vi "Initialise.vi"(8 "error in (no error)":errorcluster, 11 "SMP in":refnum<class "SMP.lvclass">) -> (0 "error out":errorcluster, 3 "SMP out":refnum<class "SMP.lvclass">)   [LabVIEW 2013, in "SMP.lvclass"]
doc: "Initialise a new SMP object. This can be used to easily implement the Pipe and Filter design pattern within a state machine. The SMP object uses a queue internally.\n\nClick on <b>Detailed help</b> for a description of the Pipe and Filter design pattern.\n\n<b>SMP in: </b>If an existing SMP object is wired to the input, it will be closed upon the successfull initialisation of the new object. If the initialisation of the new object fails, the input object will be returned unchanged."
uses:
  SMP.lvclass
  private/classData.ctl
  Data types/operation.ctl
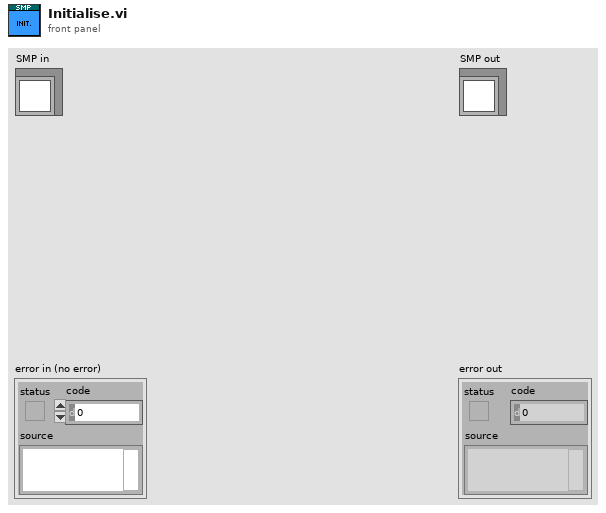
[diagram p1: front panel]
types:
  T1 = typedef "SMP.lvclass/operation.ctl" = cluster{"Name":string, "Data":variant}
  T2 = typedef "SMP.lvclass/classData.ctl" = cluster{"Q ref":refnum<queue>, "Previous data":variant, "Current pipe":T1[]}
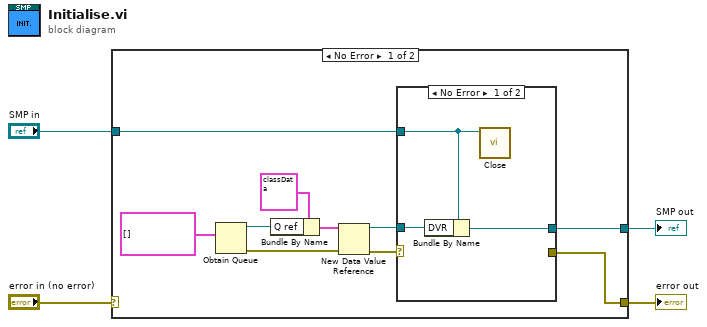
[diagram p0: block diagram]
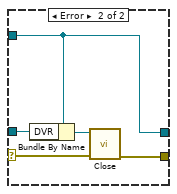
[diagram p2: hidden frame]
diagram:
  n1 = case shown="No Error" "error in (no error)" {
    selector: "error in (no error)" -> [_ w24]
    tunnel: [w5 w24] -> w3
    tunnel: [w6 w23] -> w1
    tunnel: "SMP in" -> [w8 w23]
    frame No Error {
      n2 = Obtain Queue(element data type=T1[] []) -> (queue out=w12:refnum<queue>, error out=w10:errorcluster)  [unwired: 4 in, 1 out]
      n3 = Bundle By Name(cluster=T2 {"Q ref"=refnum, "Previous data"=variant, "Current pipe"=[]} ("Class data"), "Q ref"=w12) -> (w11:T2)
      n4 = New Data Value Reference(data value=w11, error in=w10) -> (data value reference=w7:refnum<data-value>, error out=w9:errorcluster)
      n5 = case shown="No Error" w9 {
        selector: w9 -> [_ w19]
        tunnel: w8 -> [w17 w20]
        tunnel: w7 -> [w16 w22]
        tunnel: [w15 w20] -> w6
        tunnel: [_ w18] -> w5
        frame No Error {
          n6 = Bundle By Name(cluster=w17, "DVR"=w16) -> (w15:refnum<class "SMP.lvclass">)
          n7 = call "Close.vi"("SMP in"=w17) -> ()  [unwired: 10 in, 1 out]
        }
        frame Error {
          n8 = Bundle By Name(cluster=w20, "DVR"=w22) -> (w21:refnum<class "SMP.lvclass">)
          n9 = call "Close.vi"("error in (no error)"=w19, "SMP in"=w21) -> ("error out"=w18:errorcluster)  [unwired: 9 in]
        }
      }
    }
    frame Error {
    }
  }
  "error out" <- w3
  "SMP out" <- w1
